vi "Mark_StoN.vi"(1 "Marker(Low->High)":string, 2 "MarkerString":string[](array[string])) -> (5 "MarkerNumber":u32[](array[numeric]))   [LabVIEW 2016, in "ExpData.lvclass"]
uses:
  ExpData.lvclass
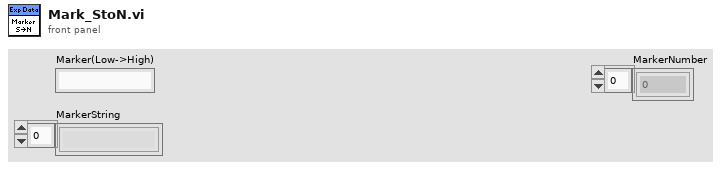
[diagram p1: front panel]
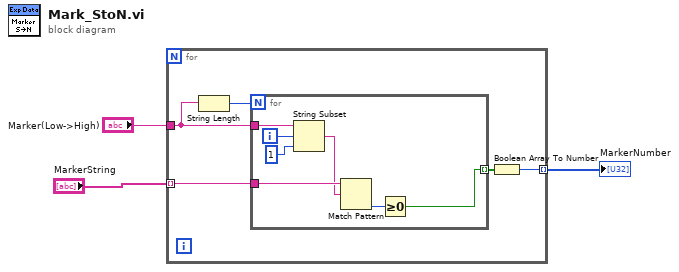
[diagram p0: block diagram]
diagram:
  n1 = for {
    tunnel: "MarkerString" -> [w6] mode=indexing
    tunnel: "Marker(Low->High)" -> [w7]
    tunnel: [w4] -> w1 mode=indexing
    n2 = String Length(string=w7) -> (length=w8:i32)
    n3 = for {
      N: w8 -> [_]
      tunnel: w7 -> [w15]
      tunnel: w6 -> [w13]
      tunnel: [w9] -> w5 mode=indexing
      i -> [w10]
      n4 = String Subset(string=w15, offset (0)=w10, length (rest)=1 ("length (rest)")) -> (substring=w12:string)
      n5 = Match Pattern(string=w13, regular expression=w12) -> (offset past match=w11:i32)  [unwired: 1 in, 3 out]
      n6 = Greater Or Equal To 0?(x=w11) -> (x >= 0?=w9:bool)
    }
    n7 = Boolean Array To Number(Boolean array=w5) -> (number=w4:u32)
  }
  "MarkerNumber" <- w1
